vi "CDMA_TxTrchCoder.vi"(8 "error in (no error)":errorcluster caption="错误输入（无错误）", 9 "coder_type":dbl, 10 "attach_crc_data":dbl[](array[numeric]), 11 "Path":path) -> (0 "error out":errorcluster caption="错误输出", 2 "tch_code_data":dbl[](array[numeric]), 3 "Path Out":path)   [LabVIEW 2015]
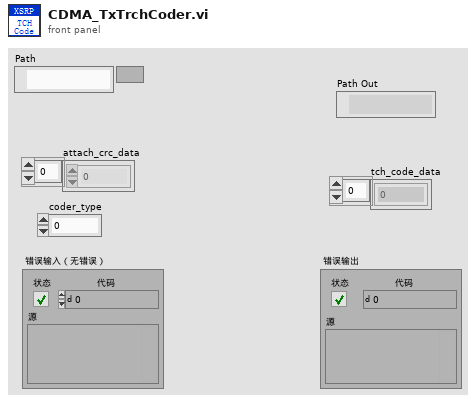
[diagram p1: front panel]
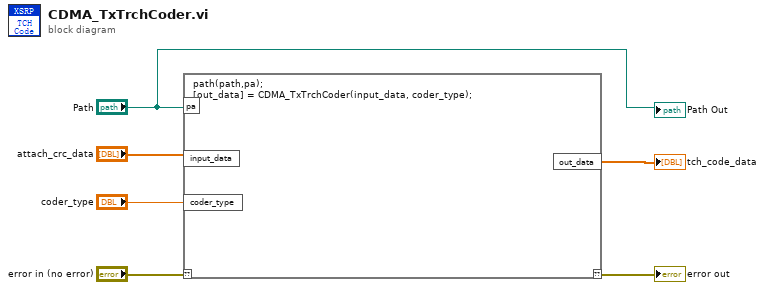
[diagram p0: block diagram]
diagram:
  n1 = script code="path(path,pa);\n[out_data] = CDMA_TxTrchCoder(input_data, coder_type);"("??"="error in (no error)", "pa"="Path", "input_data"="attach_crc_data", "coder_type"="coder_type") -> ("??"=→"error out":errorcluster, "out_data"=→"tch_code_data":dbl[])
  "Path Out" <- "Path"
